vi "PRBS64 Parallel Tx - 8 Lanes.vi"(6 "ready for output (T)":bool=TRUE, 7 "reset":bool, 11 "seed":u64[](array[numeric])=[0, 0, 0, 0, 0, 0, 0, 0]) -> (1 "output valid":bool, 3 "sequence out":u64[](array[numeric]))   [LabVIEW 2023, in "Aurora64b66b Utilities FPGA.lvlib"]
uses:
  Aurora64b66b Utilities FPGA.lvlib
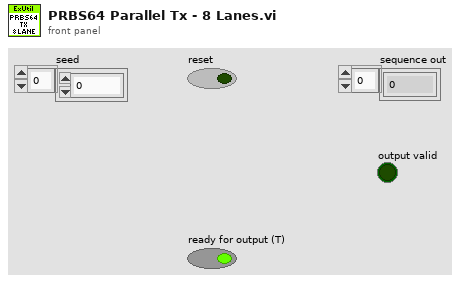
[diagram p1: front panel]
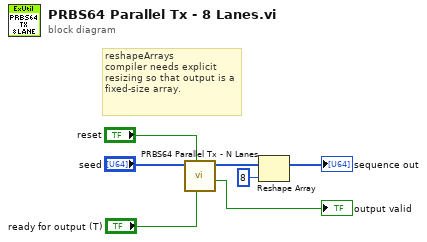
[diagram p0: block diagram]
diagram:
  # "reshapeArrays\ncompiler needs explicit resizing so that output is a fixed-size array."
  n1 = call "PRBS64 Parallel Tx - N Lanes.vi"("ready for output (T)"="ready for output (T)", "reset"="reset", "seed"="seed") -> ("output valid"=→"output valid":bool, "sequence out"=w4:u64[])  [unwired: 7 in]
  n2 = Reshape Array(w4, 8 ("dimension size")) -> (→"sequence out":u64[])
